vi "TSM SSC DCPower Configure Measurements.vi"(0 "DCPower SSC in":T2, 5 "Measurement Mode":T1 caption="Measurement Mode (Auto)", 11 "error in":errorcluster) -> (4 "DCPower SSC out":T2, 15 "error out":errorcluster)   [LabVIEW 2020]
doc: "This VI configures the measurement mode for the sessions.\n\nThe (Auto) setting automatically chooses the optimal measurement mode individually for the instrument model in each session.\n\nFrom a test time perspective Software Triggered measurements are better than using Measure Multiple, but Software Triggering isn't supported by all devices, and enabling them can make debugging in the Digital Pattern Editor more difficult.\n\nMeasure Multiple works for all devices and allows for easier debugging, but it takes longer to fetch measurements than the Software Triggered method."
uses:
  TSM/TSM SSC DCPower.ctl
  <vilib>/NI_TestStand_SemiconductorModule/NI_TestStand_Semiconductor_Module.lvlibp/PinMap/PinQueryContext/MultiplePinMultipleSessionQueryContext/MultiplePinMultipleSessionQueryContext.lvclass
  SSC DCPower/SSC DCPower.ctl
  Shared SubVIs/TSM Pin Abstraction/TSM Pin Information.ctl
  Shared SubVIs/TSM Pin Abstraction/TSM Pin Type Identifier.ctl
  Shared SubVIs/TSM Pin Abstraction/TSM Expanded Pin Information.ctl
  SSC DCPower/Measure/SSC DCPower Measurement Mode.ctl
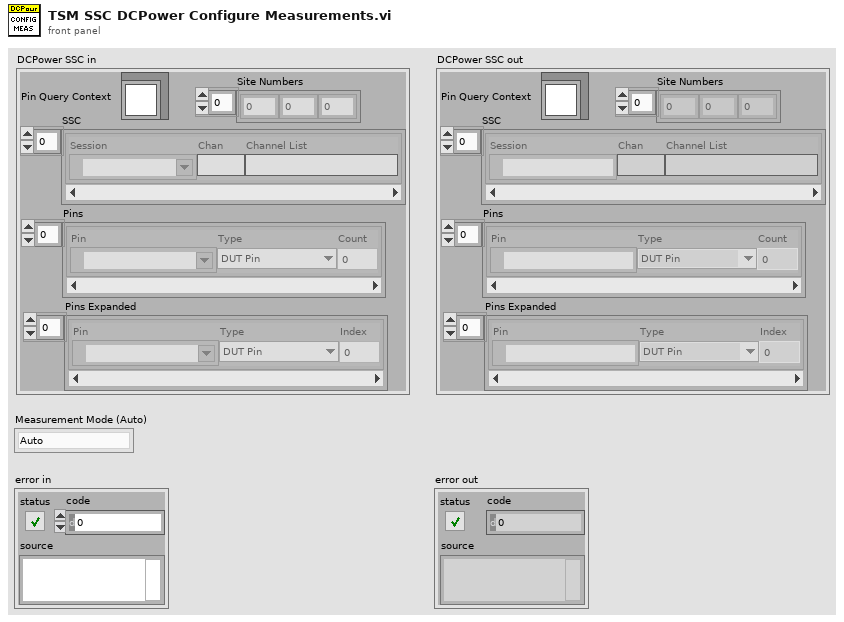
[diagram p1: front panel]
types:
  T1 = typedef "SSC DCPower Measurement Mode.ctl" = enum16{"Auto", "Measure Multiple", "Software Triggers"}
  T2 = typedef "TSM SSC DCPower.ctl" = cluster{"Pin Query Context":refnum<class "MultiplePinMultipleSessionQueryContext.lvclass">, "SSC":T3[], "Site Numbers":i32[], "Pins":T4[], "Pins Expanded":T6[]}
  T3 = typedef "SSC DCPower.ctl" = cluster{"Session":refnum<k15>, "Chan":string, "Channel List":string}
  T4 = typedef "TSM Pin Information.ctl" = cluster{"Pin":tag, "Type":T5, "Count":i32}
  T5 = typedef "TSM Pin Type Identifier.ctl" = enum8{"DUT Pin", "System Pin", "Pin Group", "Not Determined"}
  T6 = typedef "TSM Expanded Pin Information.ctl" = cluster{"Pin":tag, "Type":T5, "Index":i32}
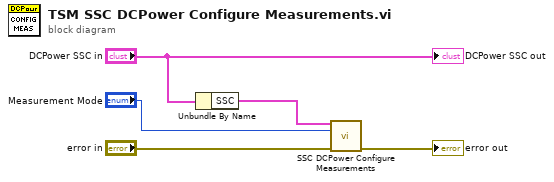
[diagram p0: block diagram]
diagram:
  n1 = Unbundle By Name("DCPower SSC in") -> ("SSC"=w2:T3[])
  n2 = call "SSC DCPower Configure Measurements.vi"("DCPower SSC in"=w2, "Measurement Mode"="Measurement Mode", "error in"="error in") -> ("error out"=→"error out":errorcluster)  [unwired: 11 in, 1 out]
  "DCPower SSC out" <- "DCPower SSC in"
